vi "Scale Cell Balance.vi"(11 "Numeric in":dbl) -> (3 "Numeric Out":dbl)   [LabVIEW 2015]
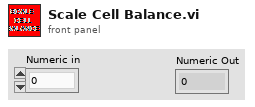
[diagram p1: front panel]
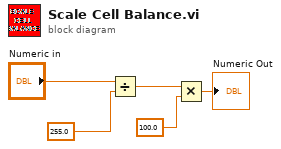
[diagram p0: block diagram]
diagram:
  n1 = Divide(x="Numeric in", y=255.0) -> (x/y=w3:dbl)
  n2 = Multiply(x=w3, y=100.0) -> (x*y=→"Numeric Out":dbl)
